vi "DSF.Shared.Configuration.Channel.Set Offset.vi"(10 "buffer offset":u64, 11 "Channel Configuration in":refnum<class "DSF.Shared.Configuration.Channel.lvclass">) -> (3 "Channel Configuration out":refnum<class "DSF.Shared.Configuration.Channel.lvclass">)   [LabVIEW 2017, in "DSF.Engine.lvlib" / "DSF.Shared.Configuration.Channel.lvclass"]
uses:
  DSF.Shared.Configuration.Channel.lvclass
  DSF.Shared.Configuration.Channel.lvclass/DSF.Shared.Configuration.Channel.ctl
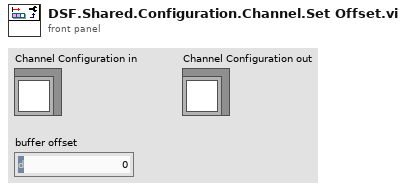
[diagram p1: front panel]
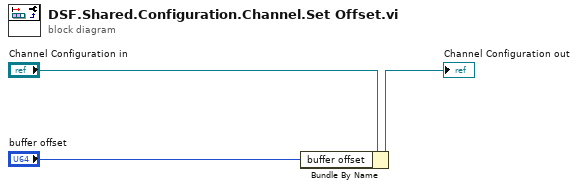
[diagram p0: block diagram]
diagram:
  n1 = Bundle By Name(cluster="Channel Configuration in", "buffer offset"="buffer offset") -> (→"Channel Configuration out":refnum<class "DSF.Shared.Configuration.Channel.lvclass">)
